vi "Digital - Perform TDR.vi"(0 "TSM context":T1) -> (15 "error out":errorcluster)   [LabVIEW 2019]
uses:
  <vilib>/NI_TestStand_SemiconductorModule/NI_TestStand_Semiconductor_Module.lvlibp/PinMap/General/SemiconductorModuleContext.ctl
  <vilib>/NI_TestStand_SemiconductorModule/NI_TestStand_Semiconductor_Module.lvlibp/PinMap/General/NIInstrumentTypeIDs.ctl
  <vilib>/NI_TestStand_SemiconductorModule/NI_TestStand_Semiconductor_Module.lvlibp
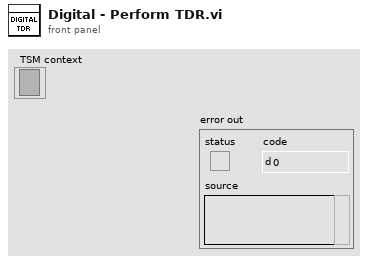
[diagram p1: front panel]
types:
  T1 = typedef "NI_TestStand_Semiconductor_Module.lvlibp/SemiconductorModuleContext.ctl" = refnum<k7>
  T2 = typedef "NI_TestStand_Semiconductor_Module.lvlibp/NIInstrumentTypeIDs.ctl" = string
  T3 = typedef "TSM SSC Digital.ctl" = cluster{"Pin Query Context":refnum<class "DigitalPatternPinQueryContext.lvclass">, "SSC":T4[], "Site Numbers":i32[], "Pins":tag[]}
  T4 = typedef "SSC Digital.ctl" = cluster{"Session":refnum<k15>, "Channel List":string, "Site List":string}
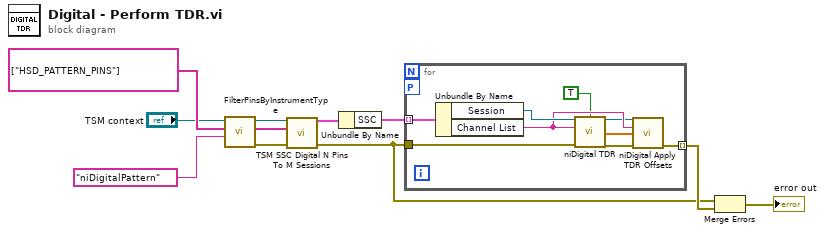
[diagram p0: block diagram]
diagram:
  n1 = call <vilib>:"FilterPinsByInstrumentType.vi"("Instrument Type Id"=T2 "niDigitalPattern", "Pins"=string[] ["HSD_PATTERN_PINS"] ("Digital"), "Semiconductor Module Context"="TSM context") -> ("error out"=w4:errorcluster, "Filtered Pins"=w6:tag[], "Semiconductor Module Context Out"=w5:T1)  [unwired: 6 in]
  n2 = call "TSM SSC Digital N Pins To M Sessions.vi"("TSM context"=w5, "Pins"=w6, "error in"=w4) -> ("Digital TSM Out"=w2:T3, "error out"=w3:errorcluster)  [unwired: 11 in]
  n3 = Unbundle By Name(w2) -> ("SSC"=w9:T4[])
  n4 = for {
    tunnel: w9 -> [w20] mode=indexing
    tunnel: w3 -> [w18]
    tunnel: [w13] -> w8 mode=indexing
    workers-P: _ -> [_]
    n5 = Unbundle By Name(w20) -> ("Session"=w19:refnum<k15>, "Channel List"=w16:string)
    n6 = call <instrlib>:"niDigital TDR.vi"("instrument handle"=w19, "apply offsets (T)"=TRUE, "channel list"=w16, "error in"=w18) -> ("instrument handle out"=w15:refnum<k15>, "offsets (s)"=w17:dbl[], "error out"=w14:errorcluster)  [unwired: 9 in]
    n7 = call <instrlib>:"niDigital Apply TDR Offsets.vi"("instrument handle"=w15, "channel list"=w16, "offsets (s)"=w17, "error in"=w14) -> ("error out"=w13:errorcluster)  [unwired: 10 in, 1 out]
  }
  n8 = Merge Errors(w3, w8) -> (→"error out":errorcluster)
